vi "ControlEvent.vi"(8 "NewValue":variant, 11 "Ctl Refnum":refnum<vi>) -> ()   [LabVIEW 2010]
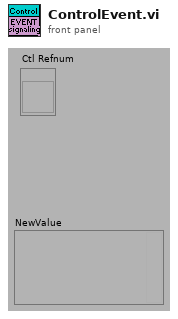
[diagram p1: front panel]
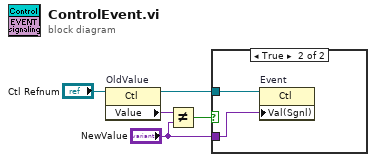
[diagram p0: block diagram]
diagram:
  n1 = property on="OldValue" class="Ctl"(reference="Ctl Refnum") -> (reference out=w4:refnum<vi>, "Value"=w3:variant)  [unwired: 1 in, 1 out]
  n2 = Not Equal?(x=w3, y="NewValue") -> (x != y?=w1:bool)
  n3 = case shown="True" w1 {
    tunnel: w4 -> [_ w7]
    tunnel: "NewValue" -> [_ w6]
    frame False {
    }
    frame True {
      n4 = property on="Event" class="Ctl"(reference=w7, "Val(Sgnl)"=w6) -> ()  [unwired: 1 in, 2 out]
    }
  }
